vi "Check FPGA Resource Manager Visualizer Status.vi"   [LabVIEW 2016, in "FPGA Addon System Explorer.lvlib"]
uses:
  Source/System Explorer/FPGA Addon System Explorer.lvlib
  <vilib>/NI VeriStand/Custom Device API/Custom Device API.lvlib
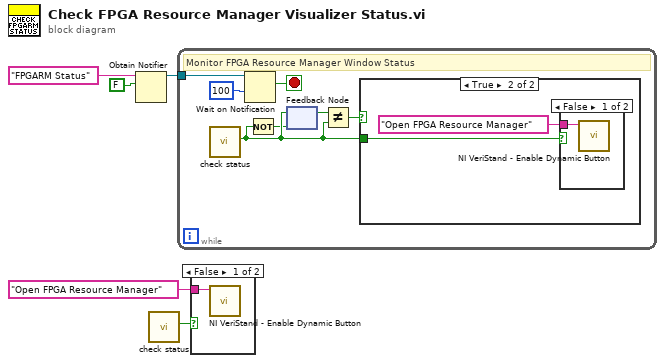
[diagram p0: block diagram]
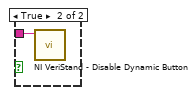
[diagram p2: hidden frame]
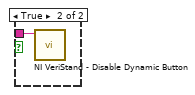
[diagram p4: hidden frame]
diagram:
  n1 = Obtain Notifier(name (unnamed)="FPGARM Status", notification data type=FALSE) -> (notifier out=w3:refnum<notifier>)  [unwired: 2 in, 2 out]
  n2 = call "check status.vi"() -> ("status"=w1:bool)  [unwired: 10 in, 1 out]
  n3 = while {
    tunnel: w3 -> [w12]
    stop <- w11 stop-if-true
    # "Monitor FPGA Resource Manager Window Status"
    n4 = call "check status.vi"() -> ("status"=w7:bool)  [unwired: 10 in, 1 out]
    n5 = Wait on Notification(notifier=w12, timeout in ms (-1)=100) -> (notification=w11:bool)  [unwired: 2 in, 3 out]
    n6 = Not(x=w7) -> (.not. x?=w6:bool)
    n7 = feedback-in #1(w7) -> ()
    n8 = feedback #1(w6) -> (w9:bool)
    n9 = Not Equal?(x=w9, y=w7) -> (x != y?=w8:bool)
    n10 = case shown="True" w8 {
      tunnel: w7 -> [_ w13]
      frame False {
      }
      frame True {
        n11 = case shown="False" w13 {
          tunnel: "Open FPGA Resource Manager" ("Button ID") -> [w15 w16]
          frame False {
            n12 = call <vilib>:"NI VeriStand - Enable Dynamic Button.vi"("Button ID"=w15) -> ()  [unwired: 10 in, 1 out]
          }
          frame True {
            n13 = call <vilib>:"NI VeriStand - Disable Dynamic Button.vi"("Button ID"=w16) -> ()  [unwired: 10 in, 1 out]
          }
        }
      }
    }
  }
  n14 = case shown="False" w1 {
    tunnel: "Open FPGA Resource Manager" ("Button ID") -> [w17 w18]
    frame False {
      n15 = call <vilib>:"NI VeriStand - Enable Dynamic Button.vi"("Button ID"=w17) -> ()  [unwired: 10 in, 1 out]
    }
    frame True {
      n16 = call <vilib>:"NI VeriStand - Disable Dynamic Button.vi"("Button ID"=w18) -> ()  [unwired: 10 in, 1 out]
    }
  }
